vi "Set Window Title Bar Icon.vi"(8 "error in (no error)":errorcluster, 10 "ICO Icon":path, 11 "VIRef":refnum<vi>) -> (0 "Error Out":errorcluster)   [LabVIEW 2023]
uses:
  user32.dll
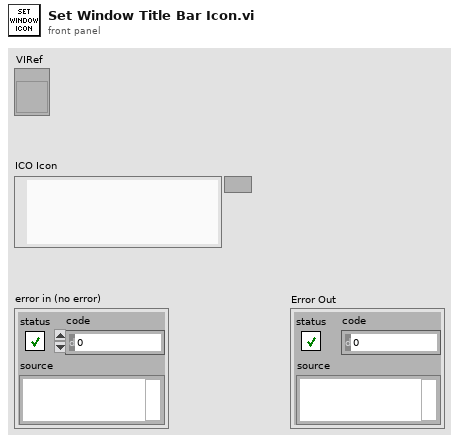
[diagram p1: front panel]
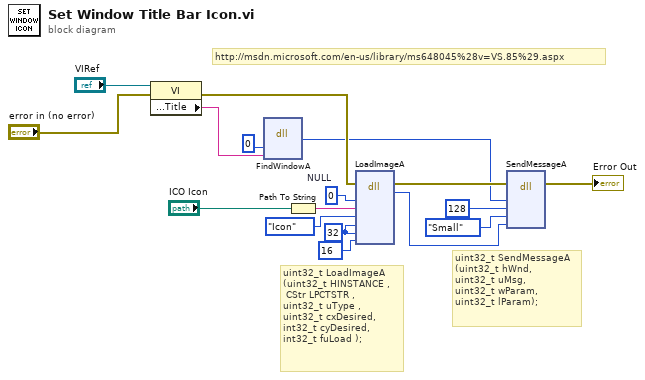
[diagram p0: block diagram]
diagram:
  w12 = u32 32 ("cxDesired")
  w11 = u32 0  # NULL
  # "uint32_t SendMessageA\n(uint32_t hWnd,\nuint32_t uMsg,\nuint32_t wParam,\nuint32_t lParam);"
  # "uint32_t LoadImageA\n(uint32_t HINSTANCE ,\n CStr LPCTSTR ,\nuint32_t uType , \nuint32_t cxDesired, \nint32_t cyDesired, \nint32_t fuLoad );"
  # "http://msdn.microsoft.com/en-us/library/ms648045%28v=VS.85%29.aspx"
  n1 = property class="VI"(reference="VIRef", error in="error in (no error)") -> (error out=w9:errorcluster, "Front Panel.Title"=w4:string)  [unwired: 1 out]
  n2 = dll-call lib="user32.dll" fn="FindWindowA" label="FindWindow"("lpszClassName"=0, "lpszWindowName"=w4) -> ("hWnd"=w2:u32)  [unwired: 5 in, 2 out]
  n3 = Path To String(path="ICO Icon") -> (string=w14:string)
  n4 = dll-call lib="user32.dll" fn="LoadImageA" label="LoadImage"(error in=w9, "HINSTANCE"=w11, "LPCTSTR"=w14, "uType"=enum16{"Bitmap", "Icon", "Cursor"}."Icon", "cxDesired"=w12, "cyDesired"=w12, "fuLoad"=16) -> (error out=w10:errorcluster, "ImageHandle"=w1:u32)  [unwired: 8 in, 1 out]
  n5 = dll-call lib="user32.dll" fn="SendMessageA" label="SendMessage"(error in=w10, "hWnd"=w2, "uMsg"=128 ("dimension size"), "wParam"=enum16{"Small", "Big"}."Small", "lParam"=w1) -> (error out=→"Error Out":errorcluster)  [unwired: 7 in, 1 out]
